vi "Module Type.vi"(11 "System Status Module in":refnum<class "System Status Module.lvclass">) -> (2 "Module Type":string)   [LabVIEW 2020, in "VolatusGUI.lvlib" / "System Status Module.lvclass"]
uses:
  System Status Module.lvclass
  System Status Module.lvclass/System Status Module.ctl
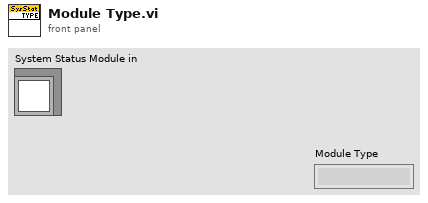
[diagram p1: front panel]
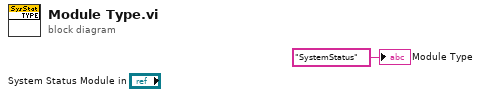
[diagram p0: block diagram]
diagram:
  "Module Type" <- "SystemStatus" ("Module Type")
